vi "GetNodeName.vi"(0 "reference in":refnum<class "PackageNode.lvclass">, 5 "error in (no error)":errorcluster) -> (14 "reference out":refnum<class "PackageNode.lvclass">, 15 "String":string, 19 "error out":errorcluster)   [LabVIEW 2014, in "PackageNode.lvclass"]
uses:
  <resource>/Framework/Providers/Open_GDS/UML/PackageNode_class/PackageNode.lvclass
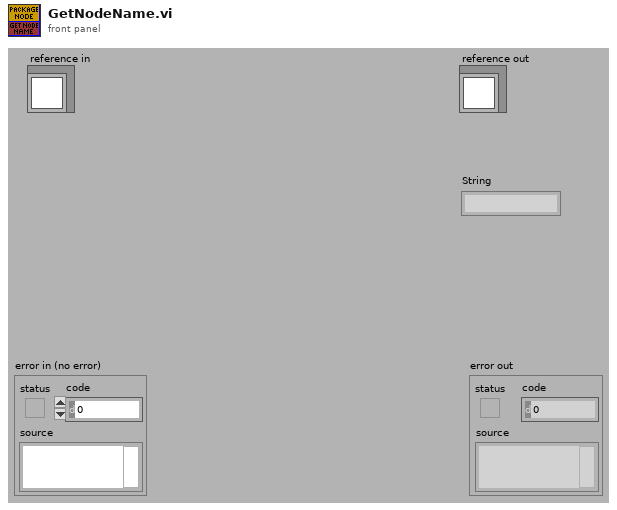
[diagram p1: front panel]
types:
  T1 = typedef "PackageNode.lvclass/ObjectAttributes.ctl" = cluster{"name":string, "contents":refnum<class "MultiLineString.lvclass">, "DEFAULT_TOP_WIDTH":i32, "DEFAULT_TOP_HEIGHT":i32, "DEFAULT_WIDTH":i32, "DEFAULT_HEIGHT":i32, "NAME_GAP":i32, "XGAP":i32, "YGAP":i32, "Collapsed":bool, "Note color":u32, "Justification":u16}
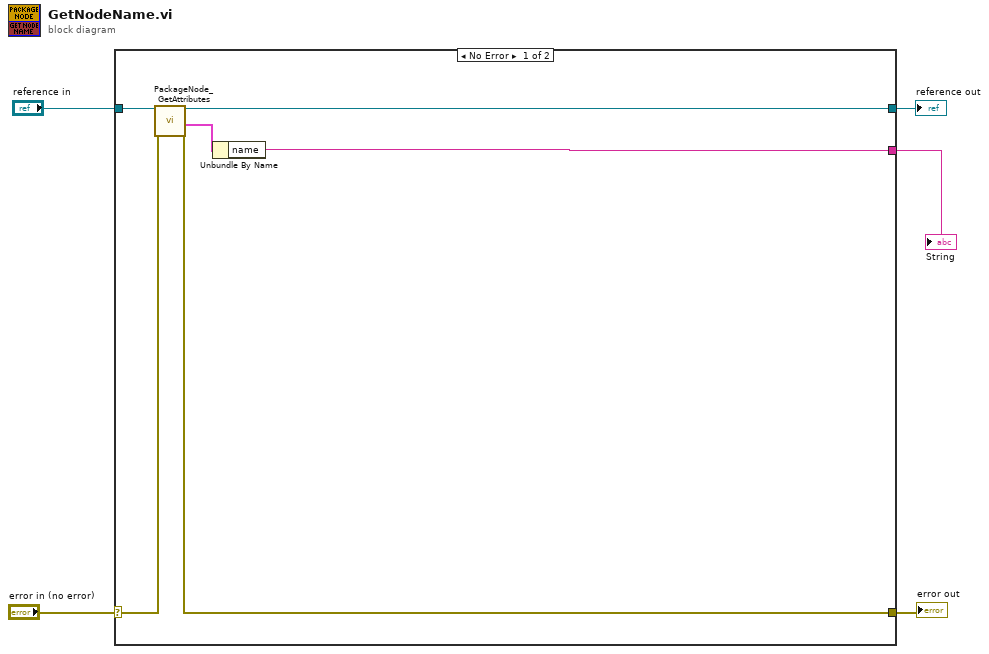
[diagram p0: block diagram]
diagram:
  n1 = case shown="No Error" "error in (no error)" {
    selector: "error in (no error)" -> [w11 w13]
    tunnel: [w10 w13] -> w4
    tunnel: [w8 w12] -> w2
    tunnel: "reference in" -> [w9 w12]
    tunnel: [w7 _] -> w1
    frame No Error {
      n2 = call <resource>:"PackageNode_GetAttributes.vi"("reference in"=w9, "error in (no error)"=w11) -> ("reference out"=w8:refnum<class "PackageNode.lvclass">, "Data"=w6:T1, "error out"=w10:errorcluster)  [unwired: 14 in, 1 out]
      n3 = Unbundle By Name(w6) -> ("name"=w7:string)
    }
    frame Error {
    }
  }
  "error out" <- w4
  "reference out" <- w2
  "String" <- w1
